vi "APEX-save_spectrum_file.vi"(0 "VISA resource input":refnum<visa-resource-name>, 5 "Trace Number":i32=1 min=1 max=6, 7 "File Name":string, 9 "File Path":string, 11 "error in (no error)":errorcluster) -> (4 "VISA resource output":refnum<visa-resource-name>, 15 "error out":errorcluster)   [LabVIEW 2020]
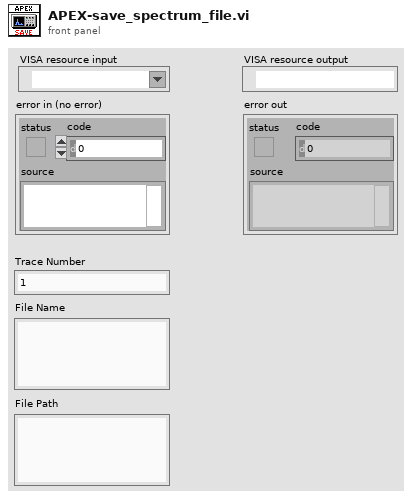
[diagram p1: front panel]
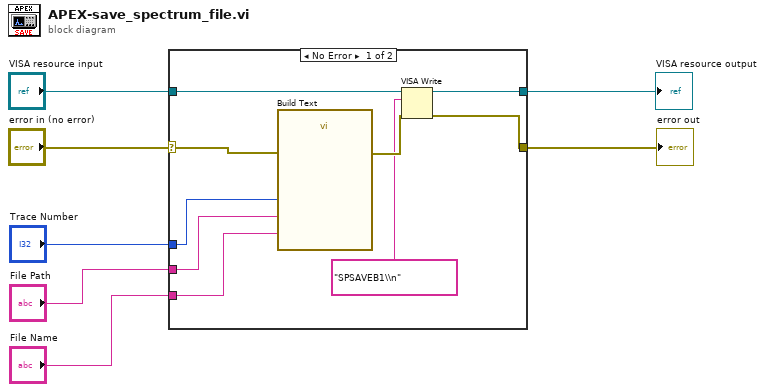
[diagram p0: block diagram]
diagram:
  n1 = case shown="No Error" "error in (no error)" {
    selector: "error in (no error)" -> [w15 w17]
    tunnel: [w13 w18] -> w2
    tunnel: "VISA resource input" -> [w16 w18]
    tunnel: [w12 w17] -> w1
    tunnel: "File Path" -> [w10 _]
    tunnel: "Trace Number" -> [w11 _]
    tunnel: "File Name" -> [w9 _]
    frame No Error {
      n2 = call "Build Text"("Trace Number"=w11, "File Path"=w10, "File Name"=w9, "error in (no error)"=w15) -> ("error out"=w14:errorcluster)  [unwired: 10 in, 1 out]
      n3 = VISA Write(VISA resource name=w16, write buffer="SPSAVEB1\\n", error in (no error)=w14) -> (VISA resource name out=w13:refnum<visa-resource-name>, error out=w12:errorcluster)  [unwired: 1 out]
    }
    frame Error {
    }
  }
  "VISA resource output" <- w2
  "error out" <- w1
